vi "Trashcan_arm.vi"(11 "Trash can arm":bool) -> (2 "Arm_Ext":bool, 3 "Arm_Down":bool)   [LabVIEW 2014]
panel:
  in  "Time_Flipper_On":i32=300
  # "THis code it to get a Can"
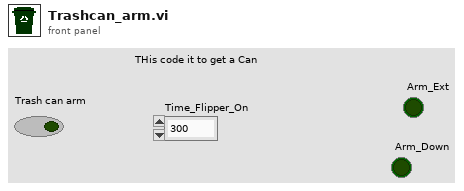
[diagram p1: front panel]
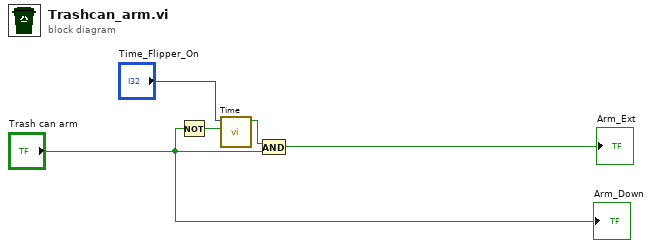
[diagram p0: block diagram]
diagram:
  n1 = Not(x="Trash can arm") -> (.not. x?=w5:bool)
  n2 = call "Time.vi"("Reset"=w5, "Time_Limit"="Time_Flipper_On") -> ("Time_Met"=w3:bool)  [unwired: 9 in]
  n3 = And(x=w3, y="Trash can arm") -> (x .and. y?=→"Arm_Ext":bool)
  "Arm_Down" <- "Trash can arm"
